vi "FindFirstFreeFIleSpace.vi"(9 "MaxSearchIndex":i32, 10 "FileSize":i32, 11 "FileData":u8[](array[numeric])) -> (1 "ValueOfFreeSpace(Size)":u8, 2 "FreeSpaceFound":bool, 3 "IndexOfFirstFreeDiscSpace":i32)   [LabVIEW 2023, in "2024_9.lvclass"]
uses:
  2024_9.lvclass
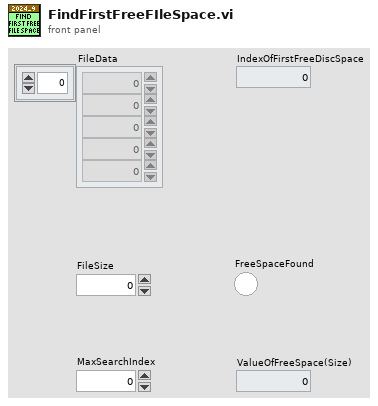
[diagram p1: front panel]
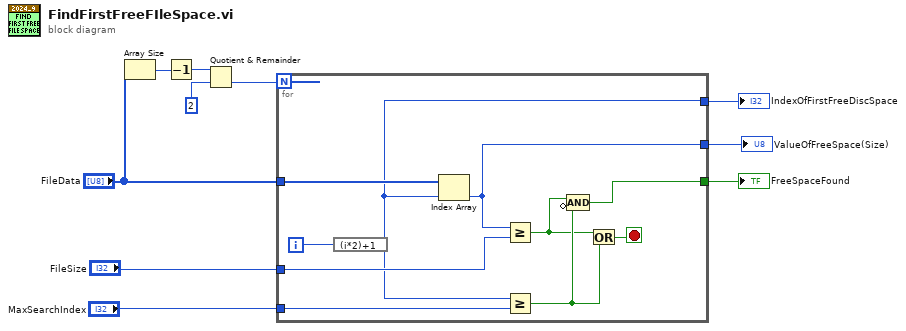
[diagram p0: block diagram]
diagram:
  n1 = Array Size(array="FileData") -> (size(s)=w9:i32)
  n2 = Decrement(x=w9) -> (x-1=w7:i32)
  n3 = Quotient & Remainder(x=w7, y=2) -> (floor(x/y)=w5:i32)  [unwired: 1 out]
  n4 = for {
    N: w5 -> [_]
    tunnel: "FileData" -> [w20]
    tunnel: [w17] -> w10
    tunnel: "FileSize" -> [w18]
    tunnel: [w11] -> w3
    tunnel: "MaxSearchIndex" -> [w16]
    tunnel: [w14] -> w1
    i -> [w19]
    stop <- w15 stop-if-true
    n5 = expression code="(i*2)+1"(w19) -> (w17:i32)
    n6 = Index Array(array=w20, index=w17) -> (element=w14:u8)
    n7 = Greater Or Equal?(x=w14, y=w18) -> (x >= y?=w12:bool)
    n8 = Greater Or Equal?(x=w17, y=w16) -> (x >= y?=w13:bool)
    n9 = Compound Arithmetic op=AND(w12, invert w13) -> (w11:bool)
    n10 = Or(x=w12, y=w13) -> (x .or. y?=w15:bool)
  }
  "IndexOfFirstFreeDiscSpace" <- w10
  "FreeSpaceFound" <- w3
  "ValueOfFreeSpace(Size)" <- w1
